vi "project-instance.vi"() -> ()   [LabVIEW 2016, in "test-find-vi-by-name.lvlib"]
uses:
  test-find-vi-by-name.lvlib
  <vilib>/addons/_JKI Toolkits/Caraya/classes/Assert/Assert Equal Value_Variant.vi
  <vilib>/addons/_JKI Toolkits/Caraya/classes/Test/Test.lvclass
  <vilib>/addons/_JKI Toolkits/Caraya/classes/Assert/Assert.lvclass
panel:
  out "error out":errorcluster
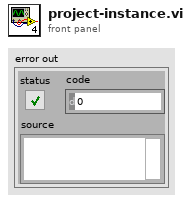
[diagram p1: front panel]
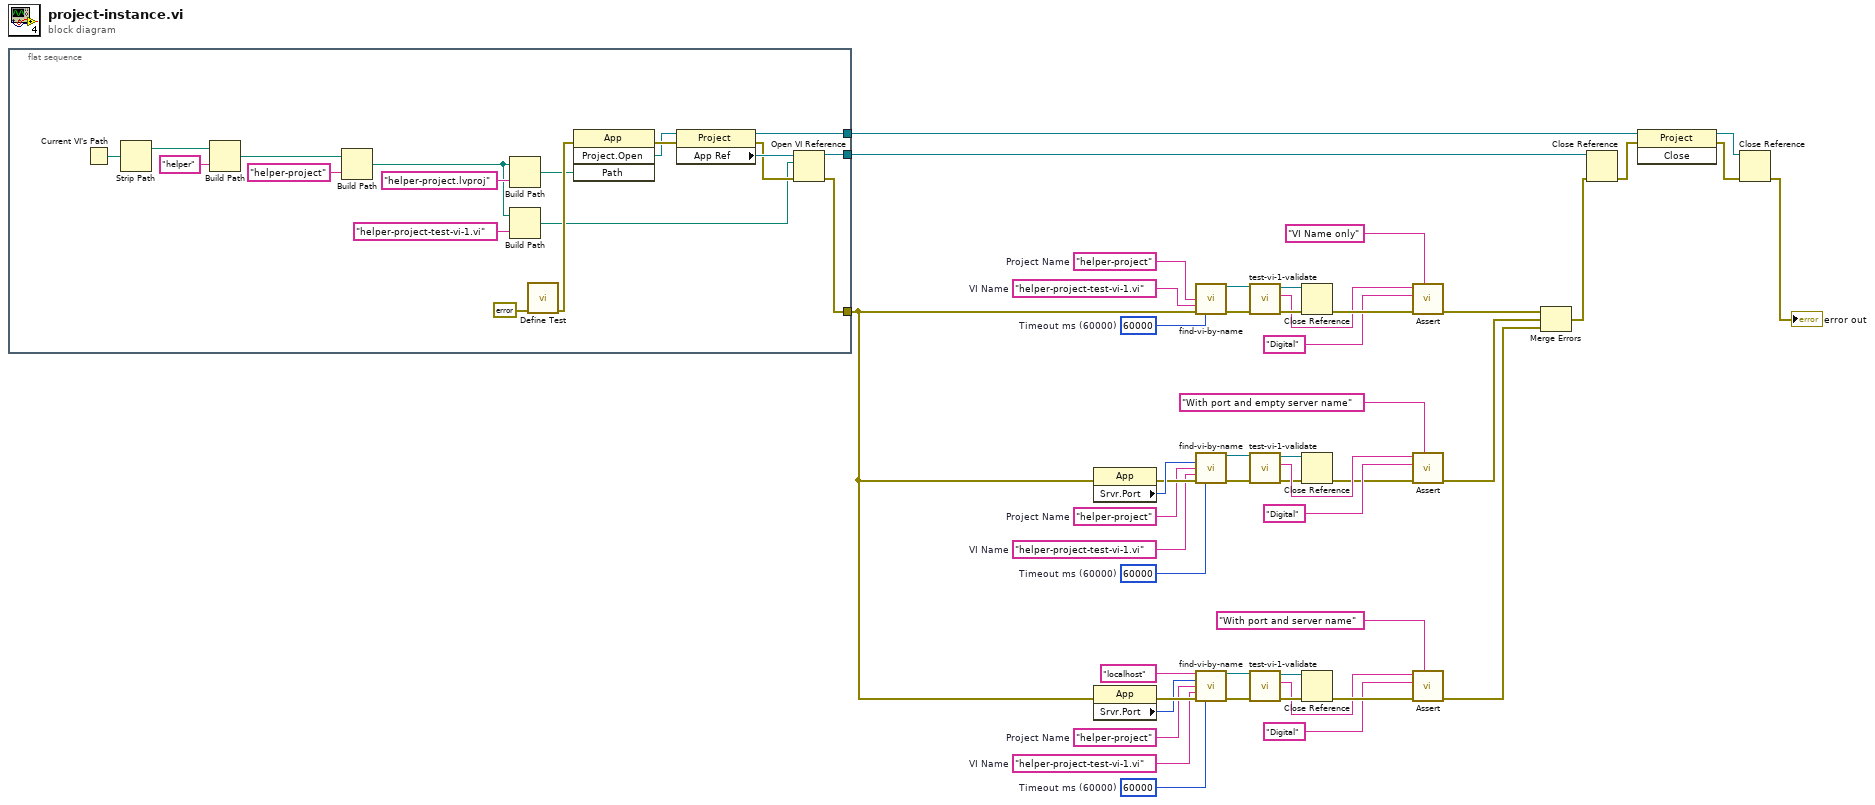
[diagram p0: block diagram]
diagram:
  w6 = "helper-project"  # Project Name
  w7 = "helper-project"  # Project Name
  w8 = "helper-project"  # Project Name
  w23 = 60000  # Timeout ms (60000)
  w9 = "helper-project-test-vi-1.vi"  # VI Name
  w33 = 60000  # Timeout ms (60000)
  w10 = "helper-project-test-vi-1.vi"  # VI Name
  w46 = 60000  # Timeout ms (60000)
  w11 = "helper-project-test-vi-1.vi"  # VI Name
  n1 = flat-sequence {
    tunnel: [w67] -> w15
    tunnel: [w66] -> w12
    tunnel: [w54] -> w5
    frame #0 {
      n2 = Current VI's Path() -> (path=w65:path)
      n3 = Strip Path(path=w65) -> (stripped path=w64:path)  [unwired: 1 out]
      n4 = Build Path(base path=w64, name or relative path="helper") -> (appended path=w62:path)
      n5 = Build Path(base path=w62, name or relative path="helper-project") -> (appended path=w50:path)
      n6 = Build Path(base path=w50, name or relative path="helper-project.lvproj") -> (appended path=w52:path)
      n7 = Build Path(base path=w50, name or relative path="helper-project-test-vi-1.vi") -> (appended path=w51:path)
      n8 = call <vilib>:"Define Test.vi"("error in (no error)"=errorcluster {"status"=FALSE, "code"=0, "source"=""}) -> ("error out"=w57:errorcluster)  [unwired: 10 in]
      n9 = invoke class="App" method="Project.Open"(error in=w57, "Path"=w52) -> (error out=w59:errorcluster, "Project:Open"=w55:refnum<vi>)  [unwired: 2 in, 2 out]
      n10 = property class="Project"(reference=w55, error in=w59) -> (reference out=w54:refnum<vi>, error out=w56:errorcluster, "App Ref"=w58:refnum<vi>)
      n11 = Open VI Reference(application reference (local)=w58, vi path=w51, error in (no error)=w56) -> (vi reference=w66:refnum<vi>, error out=w67:errorcluster)  [unwired: 3 in]
    }
  }
  n12 = property on="Property Node" class="App"(error in=w15) -> (error out=w29:errorcluster, "Srvr.Port"=w30:u32)  [unwired: 1 in, 1 out]
  n13 = property on="Property Node" class="App"(error in=w15) -> (error out=w27:errorcluster, "Srvr.Port"=w26:u32)  [unwired: 1 in, 1 out]
  n14 = call "find-vi-by-name.vi"("Project Name (\"\": Main Application Instance)"=w8, "VI Name"=w11, "error in (no error)"=w15, "Timeout ms (60000)"=w46) -> ("VI Reference"=w45:refnum<vi>, "error out"=w47:errorcluster)  [unwired: 10 in]
  n15 = call "find-vi-by-name.vi"("Port(0:Ignored)"=w30, "Project Name (\"\": Main Application Instance)"=w7, "VI Name"=w10, "error in (no error)"=w29, "Timeout ms (60000)"=w33) -> ("VI Reference"=w34:refnum<vi>, "error out"=w32:errorcluster)  [unwired: 9 in]
  n16 = call "find-vi-by-name.vi"("Service Name (\"\":localhost)"="localhost" ("Service Name (\"\":localhost)"), "Port(0:Ignored)"=w26, "Project Name (\"\": Main Application Instance)"=w6, "VI Name"=w9, "error in (no error)"=w27, "Timeout ms (60000)"=w23) -> ("VI Reference"=w22:refnum<vi>, "error out"=w24:errorcluster)  [unwired: 8 in]
  n17 = call "test-vi-1-validate.vi"("error in (no error)"=w47, "VI in"=w45) -> ("error out"=w44:errorcluster, "ClassName"=w41:string, "VI out"=w42:refnum<vi>)  [unwired: 7 in]
  n18 = call "test-vi-1-validate.vi"("error in (no error)"=w32, "VI in"=w34) -> ("error out"=w35:errorcluster, "ClassName"=w38:string, "VI out"=w37:refnum<vi>)  [unwired: 7 in]
  n19 = call "test-vi-1-validate.vi"("error in (no error)"=w24, "VI in"=w22) -> ("error out"=w21:errorcluster, "ClassName"=w18:string, "VI out"=w19:refnum<vi>)  [unwired: 7 in]
  n20 = Close Reference(reference=w42, error in (no error)=w44) -> (error out=w43:errorcluster)
  n21 = Close Reference(reference=w37, error in (no error)=w35) -> (error out=w36:errorcluster)
  n22 = Close Reference(reference=w19, error in (no error)=w21) -> (error out=w20:errorcluster)
  n23 = call-poly <vilib>:"Assert.vi"("Label"="VI Name only" ("Label (VI Title)"), "error in (no error)"=w43, "Y"="Digital" ("Class Name"), "X"=w41) -> ("error out"=w48:errorcluster)  [unwired: 7 in]
  n24 = call-poly <vilib>:"Assert.vi"("Label"="With port and empty server name" ("Label (VI Title)"), "error in (no error)"=w36, "Y"="Digital" ("Class Name"), "X"=w38) -> ("error out"=w28:errorcluster)  [unwired: 7 in]
  n25 = call-poly <vilib>:"Assert.vi"("Label"="With port and server name" ("Label (VI Title)"), "error in (no error)"=w20, "Y"="Digital" ("Class Name"), "X"=w18) -> ("error out"=w16:errorcluster)  [unwired: 7 in]
  n26 = Merge Errors(w48, w28, w16) -> (w13:errorcluster)
  n27 = Close Reference(reference=w12, error in (no error)=w13) -> (error out=w4:errorcluster)
  n28 = invoke class="Project" method="Close"(reference=w5, error in=w4) -> (reference out=w2:refnum<vi>, error out=w3:errorcluster)  [unwired: 1 in, 1 out]
  n29 = Close Reference(reference=w2, error in (no error)=w3) -> (error out=→"error out":errorcluster)
